vi "DestroyPublicEvents.vi"(8 "error in (no error)":errorcluster, 11 "Setting Database":refnum<class "Setting Database.lvclass">) -> (0 "error out":errorcluster, 3 "Setting Database out":refnum<class "Setting Database.lvclass">)   [LabVIEW 2019, in "Setting Database.lvclass"]
doc: "JKI State Machine Objects (SMO) 1.0.0.5\nJKI - JKI\nCopyright (c) 2016, JKI"
uses:
  Setting Database.lvclass
  <vilib>/JKI/JKI SMO/SMO/SMO.lvclass
panel:
  # "For instructions on how to use the JKI State Machine Objects, examples and video tutorials, visit:\nhttp://jki.net/state-machine-objects/\n\nJKI State Machine Objects™\nhttp://jki.net/state-machine-objects/\nCopyright (C) 2005-2015, JKI <info@jki.net>\nALL RIGHTS RESERVED"
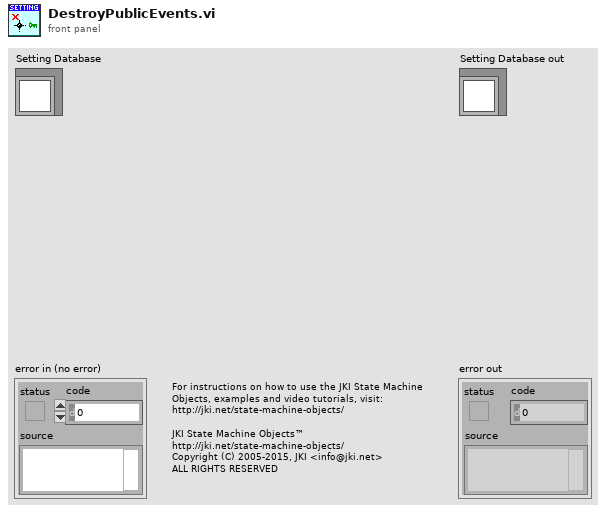
[diagram p1: front panel]
types:
  T1 = typedef "Setting Database.lvclass/PublicEvents--Cluster.ctl" = cluster{"NewActivePath":refnum<user-event>, "PathsUpdated":refnum<user-event>, "RectanglesUpdated":refnum<user-event>, "NewActiveRectangle":refnum<user-event>, "NewActiveFunnel":refnum<user-event>, "FunnelsUpdated":refnum<user-event>, "NewActiveDot":refnum<user-event>, "DotsUpdated":refnum<user-event>}
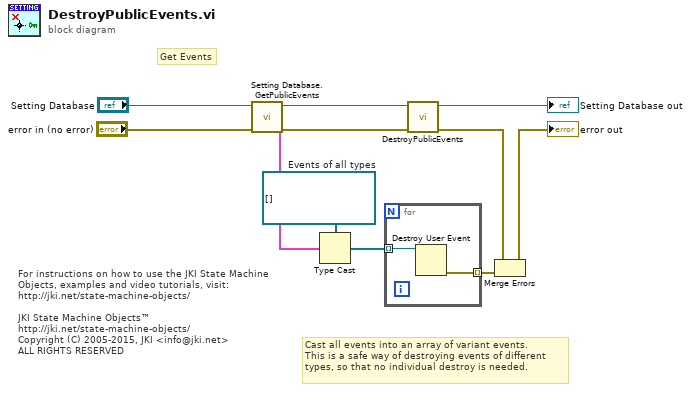
[diagram p0: block diagram]
diagram:
  w7 = refnum<user-event>[] []  # Events of all types
  # "Get Events"
  # "For instructions on how to use the JKI State Machine Objects, examples and video tutorials, visit:\nhttp://jki.net/state-machine-objects/\n\nJKI State Machine Objects™\nhttp://jki.net/state-machine-objects/\nCopyright (C) 2005-2015, JKI <info@jki.net>\nALL RIGHTS RESERVED"
  # "Cast all events into an array of variant events.\nThis is a safe way of destroying events of different\ntypes, so that no individual destroy is needed."
  n1 = call "Setting Database.GetPublicEvents.vi"("error in (no error)"="error in (no error)", "Setting Database"="Setting Database") -> ("error out"=w4:errorcluster, "Public Events"=w1:T1, "Setting Database out"=w3:refnum<class "Setting Database.lvclass">)  [unwired: 7 in]
  n2 = Type Cast(type=w7, x=w1) -> (*(type *) &x=w8:refnum<user-event>[])
  n3 = for {
    tunnel: w8 -> [w13] mode=indexing
    tunnel: [w12] -> w6 mode=indexing
    n4 = Destroy User Event(user event=w13) -> (error out=w12:errorcluster)  [unwired: 1 in]
  }
  n5 = call-parent "DestroyPublicEvents.vi"("error in (no error)"=w4, "SMO"=w3) -> ("error out"=w10:errorcluster, "SMO out"=→"Setting Database out":refnum<class "Setting Database.lvclass">)  [unwired: 8 in]
  n6 = Merge Errors(w10, w6) -> (→"error out":errorcluster)
